vi "Simulate TCP client.vi"() -> ()   [LabVIEW 2015]
panel:
  out "data out":string
  out "error out 2":errorcluster
  out "error out":errorcluster
  in  "data send":string
  in  "stop":bool
  in  "send":bool
  in  "remote port or service name":u16
  in  "address":string
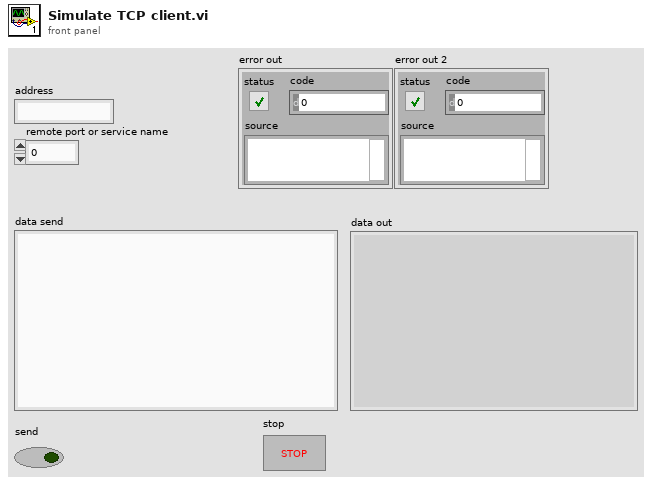
[diagram p1: front panel]
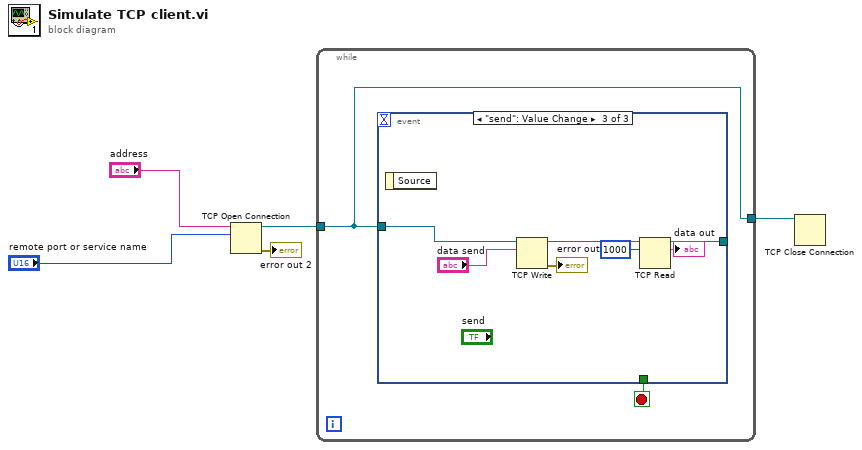
[diagram p0: block diagram]
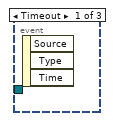
[diagram p2: hidden frame]
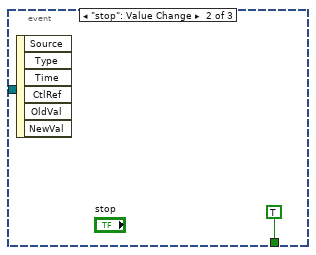
[diagram p3: hidden frame]
diagram:
  n1 = TCP Open Connection(address="address", remote port or service name="remote port or service name") -> (connection ID=w3:refnum<k5>, error out=→"error out 2":errorcluster)  [unwired: 3 in]
  n2 = while {
    tunnel: w3 -> [w6]
    tunnel: [w6] -> w2
    stop <- w7 stop-if-true
    n3 = event shown="[2] \"send\": Value Change" {
      selector: _ -> [_ _ _]
      dyn-events: _ -> [_ _ _]
      timeout: _ -> [_ _ _]
      tunnel: [_ TRUE _] -> w7
      tunnel: w6 -> [_ _ w15]
      tunnel: [_ _ w11] -> _
      event Timeout {
        n4 = event-data() -> ()  [unwired: 1 in, 3 out]
      }
      event "stop": Value Change {
        n5 = event-data() -> ()  [unwired: 1 in, 6 out]
      }
      event "send": Value Change {
        n6 = event-data() -> ()  [unwired: 1 in, 1 out]
        n7 = TCP Write(connection ID=w15, data in="data send") -> (connection ID out=w12:refnum<k5>, error out=→"error out":errorcluster)  [unwired: 2 in, 1 out]
        n8 = TCP Read(connection ID=w12, bytes to read=1000) -> (connection ID out=w11:refnum<k5>, data out=→"data out":string)  [unwired: 3 in, 1 out]
      }
    }
  }
  n9 = TCP Close Connection(connection ID=w2) -> ()  [unwired: 2 in, 2 out]
